vi "less10thanSD.vi"(1 "Array In":dbl[](array[numeric])) -> (0 "Array In out":dbl[](array[numeric]))   [LabVIEW 2015]
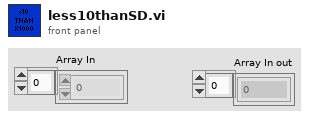
[diagram p1: front panel]
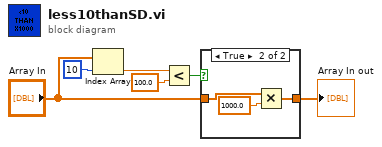
[diagram p0: block diagram]
diagram:
  n1 = Index Array(array="Array In", index=10) -> (element=w5:dbl)
  n2 = Less?(x=w5, y=100.0) -> (x < y?=w3:bool)
  n3 = case shown="True" w3 {
    tunnel: [w7 w8] -> w2
    tunnel: "Array In" -> [w7 w10]
    frame False {
    }
    frame True {
      n4 = Multiply(x=w10, y=1000.0 ("Numeric")) -> (x*y=w8:dbl[])
    }
  }
  "Array In out" <- w2
